vi "FRC Classification Example.vi"() -> ()   [LabVIEW 2025]
uses:
  <vilib>/Rock Robotics/WPI/Camera/WPI_CameraSettings Read MJPG.ctl
  <vilib>/Rock Robotics/WPI/Camera/WPI_CameraImageSize.ctl
  Vision Support Code/Camera Types.ctl
  <vilib>/vision/NI_Vision_Development_Module.lvlib
panel:
  in  "score limit":sgl
  in  "Limit Tests?":bool=TRUE
  in  "Camera Type":T1=enum."MS HD3000 square"
  in  "Image Path":path=path "Sample Images/KicoffFilmingVision"
  in  "image files":string[](array[string])
  in  "Aspect Fudge Factor":dbl=1.0
  out "Detected Targets":T2(array[cluster]) {"Normalized Rect"."Numeric 5" format="%#_2g"; "Normalized Rect"."Numeric 3" format="%#_2g"; "Normalized Rect"."Numeric 2" format="%#_2g"; "Normalized Rect"."Numeric" format="%#_2g"}
  in  "Score Threshold":dbl=75.0
  in  "Source":enum32{"Files", "Camera"}(tab)
  in  "Images":i32(listbox)
  in  "Folder Location":path=path "Sample Images/Real Tower"
  in  "Camera Settings":T3={"fps"=20, "compression"=30, "Image Size"=enum."320x240", "Config Shown"=FALSE}
  in  "Camera Address":string="USB 1"
  in  "Annotate":bool=TRUE
  out "ms to process":u32
  out "Sorted Scores":T5(array[cluster]) {"Moment Factor" format="%#_3g"; "L" format="%#_3g"; "Area to CH" format="%#_3g"; "X" format="%#_3g"; "Y" format="%#_3g"}
  in  "LED Color":T6={"Hue"={86.68604567358754, 144.18771039657545}, "Sat"={97.14285714285715, 255.0}, "Val"={39.46428571428572, 255.0}} {"Hue" scale=0.0..255.0 scale format="%#_3g"}
  out "Masked":T7(plugin-control)
  out "Original Image":T7(plugin-control)
  # "Instructions:\nUse Source to select image files from a directory, or use a USB or IP camera connected to your laptop.\nUse LED Color to threshold and build particles. Adjust HSV values to improve masking.\nAnnotations draw a rectangle around \"good\" particles with scores from top to bottom."
  # "Aspect Ratio"
  # "Density Profile"
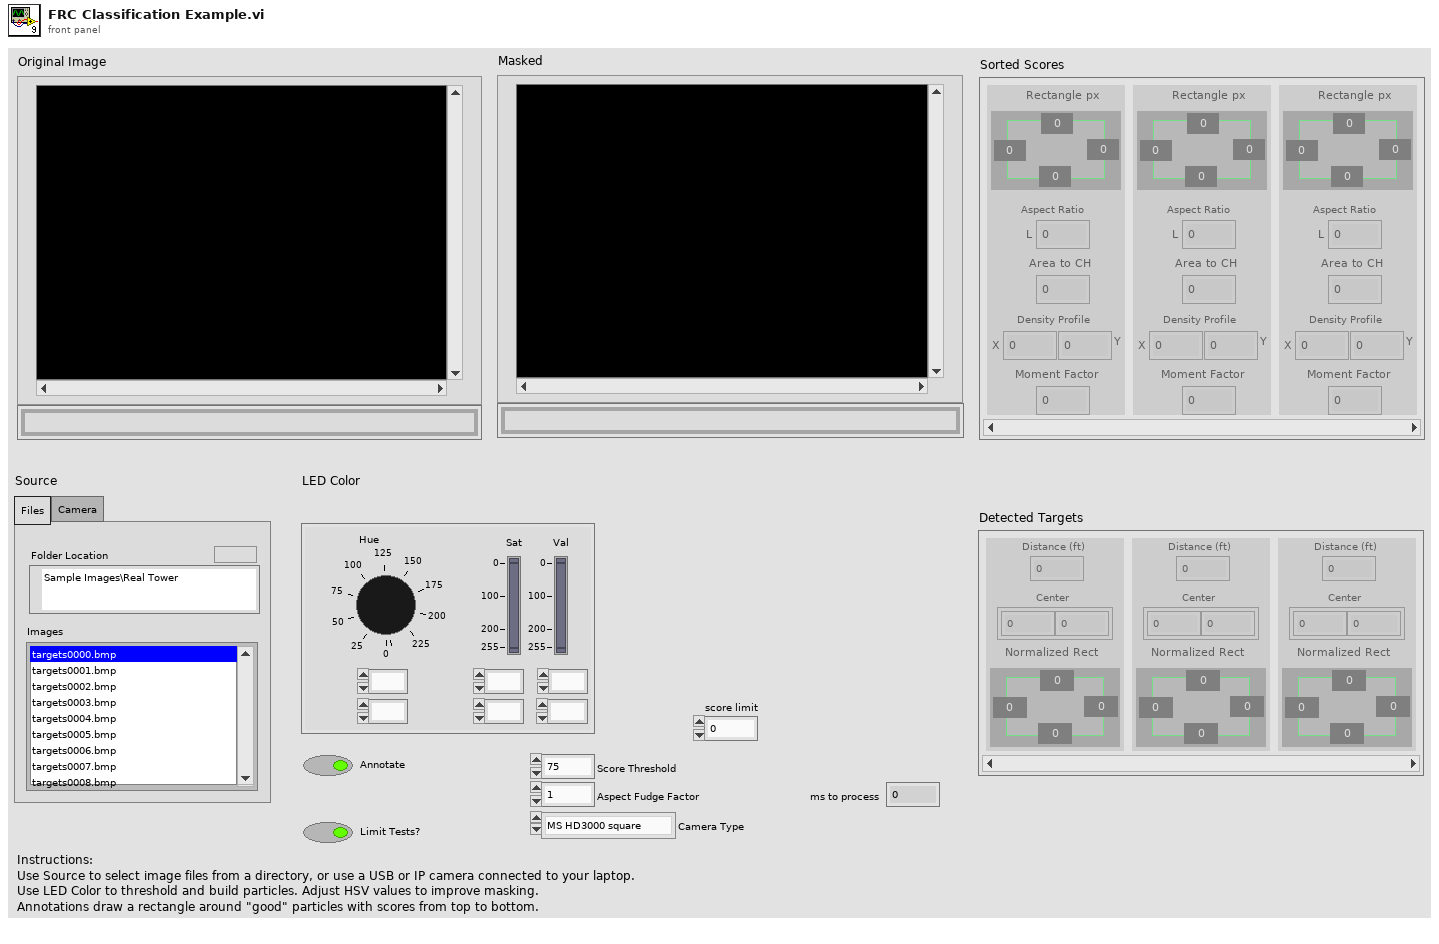
[diagram p1: front panel]
types:
  T1 = typedef "Camera Types.ctl" = enum16{"206", "1011", "1013", "MS HD3000 square", "MS HD3000 640x480"}
  T2 = cluster{"Distance (ft)":dbl, "Center":cluster{dbl, dbl}, "Normalized Rect":cluster{"Numeric":dbl, "Numeric 2":dbl, "Numeric 3":dbl, "Numeric 5":dbl}}[]
  T3 = typedef "WPI_CameraSettings Read MJPG.ctl" = cluster{"fps":i32, "compression":i32, "Image Size":T4, "Config Shown":bool}
  T4 = typedef "WPI_CameraImageSize.ctl" = enum16{"640x480", "320x240", "160x120", "Custom"}
  T5 = cluster{"Rectangle px":cluster{"Numeric":dbl, "Numeric 2":dbl, "Numeric 3":dbl, "Numeric 5":dbl}, "L":dbl, "Area to CH":dbl, "X":dbl, "Y":dbl, "Moment Factor":dbl}[]
  T6 = cluster{"Hue":cluster{dbl, dbl}, "Sat":cluster{dbl, dbl}, "Val":cluster{dbl, dbl}}
  T7 = typedef "IMAQ Image.ctl" = refnum<image>
  T8 = cluster{"Numeric":dbl, "Numeric":dbl, "Numeric":dbl, "Numeric":dbl, dbl}
  T9 = typedef "Image Type" = u32
  T10 = typedef "Particle Parameters" = i32
  T11 = typedef "IMAQ Classifier Session.ctl" = refnum<k1>
  T12 = typedef "ROI Descriptor" = cluster{"Global Rectangle":i32[], "Contours":cluster{"ID":enum32{"External", "Internal"}, "Type":u32, "Coordinates":i32[]}[]}
  T13 = cluster{"Classification Score":sgl, "Identification Score":sgl}
  T14 = cluster{"Numeric":dbl, "Numeric":dbl, "Numeric":dbl, "Numeric":dbl}
  T15 = cluster{"Rectangle":cluster{"Numeric":dbl, "Numeric 2":dbl, "Numeric 3":dbl, "Numeric 5":dbl}, "L":dbl, "Area to CH":dbl, "X":dbl, "Y":dbl, "Moment Factor":dbl}[]
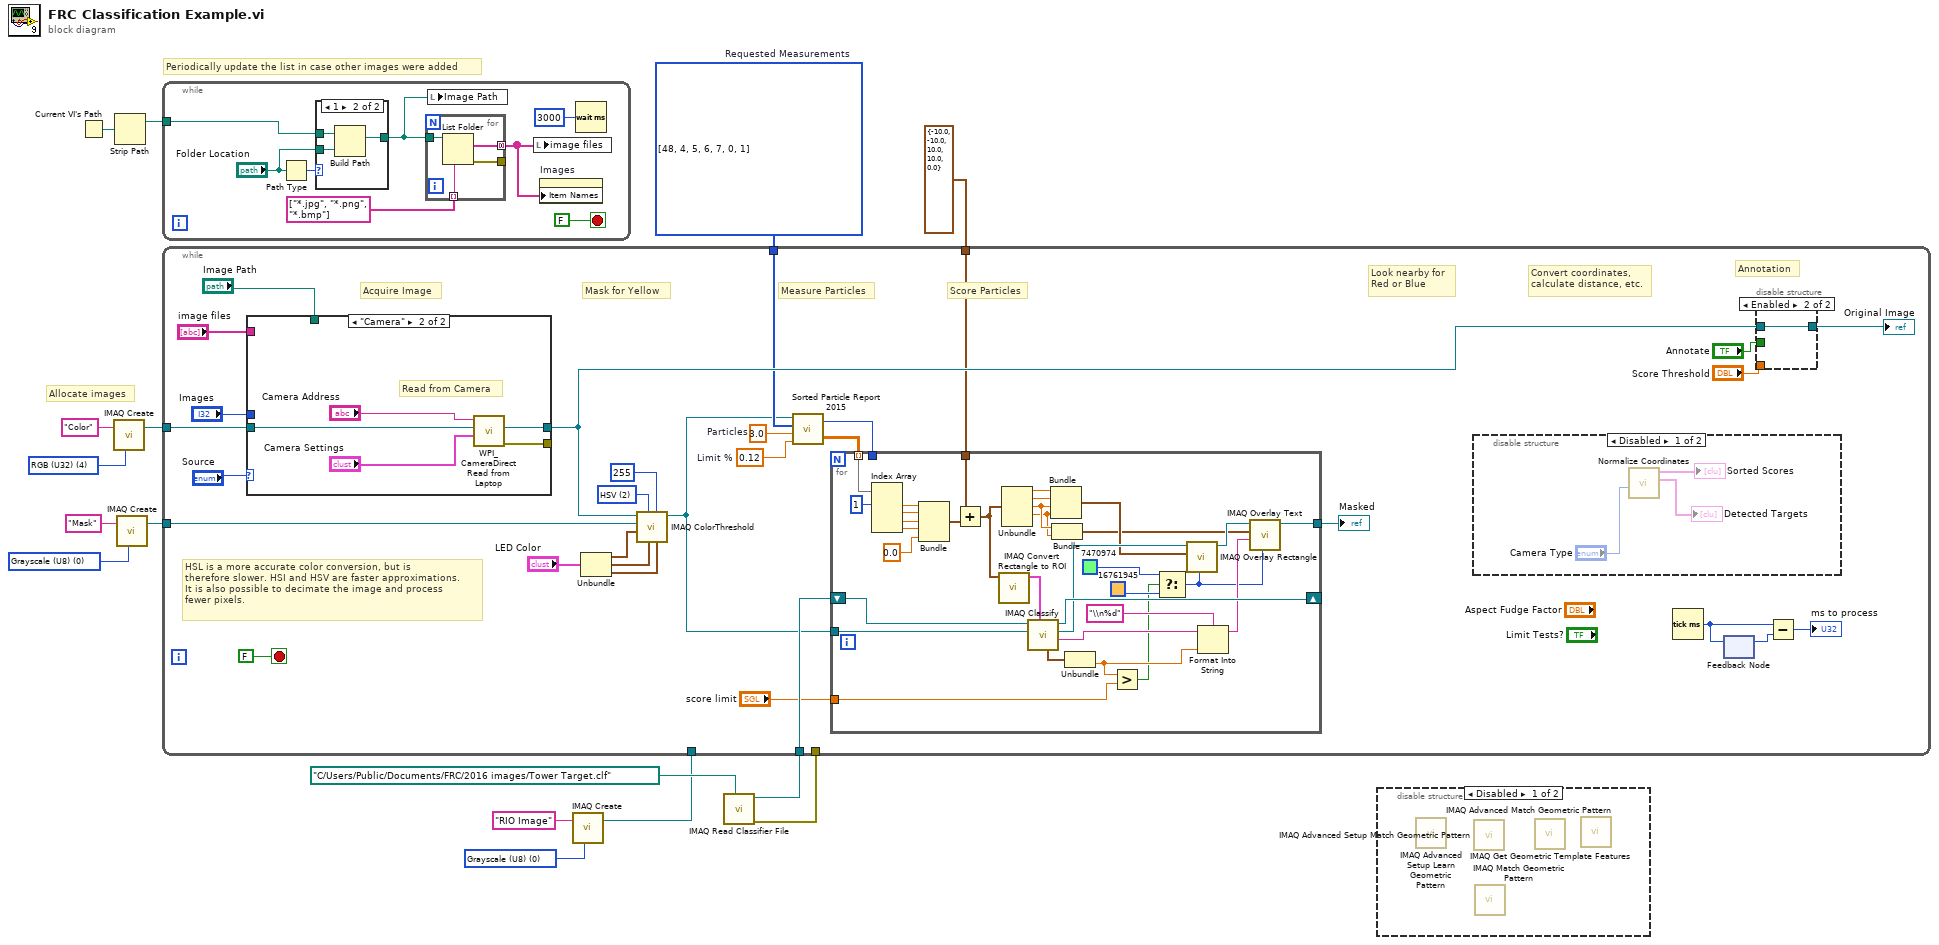
[diagram p0: block diagram]
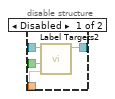
[diagram p4: hidden frame]
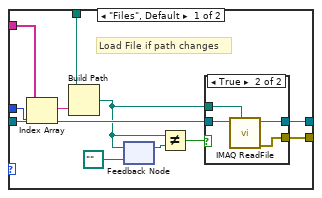
[diagram p6: hidden frame]
diagram:
  w4 = T9 0 items=["Grayscale (U8)", "Grayscale (I16)", "Grayscale (SGL)", "Complex (CSG)", "RGB (U32)", "HSL (U32)", "RGB (U64)", "Grayscale (U16)"] ("Image Type")
  w10 = T10[] [48, 4, 5, 6, 7, 0, 1] items=["Center of Mass X", "Center of Mass Y", "First Pixel X", "First Pixel Y", "Bounding Rect Left", "Bounding Rect Top", "Bounding Rect Right", "Bounding Rect Bottom", "Max Feret Diameter Start X", "Max Feret Diameter Start Y", "Max Feret Diameter End X", "Max Feret Diameter End Y", "Max Horiz. Segment Length Left", "Max Horiz. Segment Length Right", "Max Horiz. Segment Length Row", "-", "Bounding Rect Width", "Bounding Rect Height", "Bounding Rect Diagonal", "Perimeter", "Convex Hull Perimeter", "Holes' Perimeter", "Max Feret Diameter", "Equivalent Ellipse Major Axis", "Equivalent Ellipse Minor Axis", "Equivalent Ellipse Minor Axis (Feret)", "Equivalent Rect Long Side", "Equivalent Rect Short Side", "Equivalent Rect Diagonal", "Equivalent Rect Short Side (Feret)", "Average Horiz. Segment Length", "Average Vert. Segment Length", "Hydraulic Radius", "Waddel Disk Diameter", "-", "Area", "Holes' Area", "Particle & Holes' Area", "Convex Hull Area", "Image Area", "-", "Number of Holes", "Number of Horiz. Segments", "Number of Vert. Segments", "-", "Orientation", "Max Feret Diameter Orientation", "-", "% Area/Image Area", "% Area/(Particle & Holes' Area)", "Ratio of Equivalent Ellipse Axes", "Ratio of Equivalent Rect Sides", "-", "Elongation Factor", "Compactness Factor", "Heywood Circularity Factor", "Type Factor", "-", "Sum X", "Sum Y", "Sum XX", "Sum XY", "Sum YY", "Sum XXX", "Sum XXY", "Sum XYY", "Sum YYY", "-", "Moment of Inertia XX", "Moment of Inertia XY", "Moment of Inertia YY", "Moment of Inertia XXX", "Moment of Inertia XXY", "Moment of Inertia XYY", "Moment of Inertia YYY", "Norm. Moment of Inertia XX", "Norm. Moment of Inertia XY", "Norm. Moment of Inertia YY", "Norm. Moment of Inertia XXX", "Norm. Moment of Inertia XXY", "Norm. Moment of Inertia XYY", "Norm. Moment of Inertia YYY", "Hu Moment 1", "Hu Moment 2", "Hu Moment 3", "Hu Moment 4", "Hu Moment 5", "Hu Moment 6", "Hu Moment 7"]  # Requested Measurements
  w13 = T9 0 items=["Grayscale (U8)", "Grayscale (I16)", "Grayscale (SGL)", "Complex (CSG)", "RGB (U32)", "HSL (U32)", "RGB (U64)", "Grayscale (U16)"] ("Image Type")
  w15 = T9 4 items=["Grayscale (U8)", "Grayscale (I16)", "Grayscale (SGL)", "Complex (CSG)", "RGB (U32)", "HSL (U32)", "RGB (U64)", "Grayscale (U16)"] ("Image Type")
  # "Periodically update the list in case other images were added"
  # "Allocate images"
  n1 = Current VI's Path() -> (path=w9:path)
  n2 = call "IMAQ Create"("Image Name"="Color", "Image Type"=w15) -> ("New Image"=w14:T7)  [unwired: 2 in, 2 out]
  n3 = Strip Path(path=w9) -> (stripped path=w8:path)  [unwired: 1 out]
  n4 = call "IMAQ Create"("Image Name"="Mask", "Image Type"=w13) -> ("New Image"=w11:T7)  [unwired: 2 in, 2 out]
  n5 = while {
    tunnel: w8 -> [w19]
    stop <- FALSE stop-if-true
    n6 = Path Type(1:"Folder Location") -> (0:w21:i16)
    n7 = case shown="1" w21 {
      tunnel: "Folder Location" -> [w25 w28]
      tunnel: [w25 w26] -> w18
      tunnel: w19 -> [_ w27]
      frame 0, Default {
      }
      frame 1 {
        n8 = Build Path(base path=w27, name or relative path=w28) -> (appended path=w26:path)
      }
    }
    n9 = for {
      tunnel: [w32] -> w22 mode=concatenating
      tunnel: w18 -> [w31]
      tunnel: string[] ["*.jpg", "*.png", "*.bmp"] -> [w30] mode=indexing
      tunnel: [w29] -> _
      n10 = List Folder(path=w31, pattern=w30) -> (filenames=w32:string[], error out=w29:errorcluster)  [unwired: 2 in, 2 out]
    }
    n11 = local write "Image Path"(w18) -> ()
    n12 = local write "image files"(w22) -> ()
    n13 = property on="Images" class="LstBox (strict)"("Item Names"=w22) -> ()  [unwired: 2 in, 2 out]
    n14 = Wait (ms)(milliseconds to wait=u32 3000) -> ()  [unwired: 1 out]
  }
  n15 = call "IMAQ Create"("Image Name"="RIO Image", "Image Type"=w4) -> ("New Image"=w3:T7)  [unwired: 2 in, 2 out]
  n16 = call "IMAQ Read Classifier File"("File Path"=path "C:/Users/Public/Documents/FRC/2016 images/Tower Target.clf") -> ("error out"=w2:errorcluster, "Classifier Session"=w6:T11)  [unwired: 6 in, 3 out]
  n17 = while {
    tunnel: w14 -> [w61]
    tunnel: w11 -> [w60]
    tunnel: w10 -> [w41]
    tunnel: w6 -> [w44]
    tunnel: w3 -> [_]
    tunnel: w2 -> [_]
    tunnel: T8 {"Numeric"=-10.0, "Numeric"=-10.0, "Numeric"=10.0, "Numeric"=10.0, 0.0} ("x") -> [w38]
    stop <- FALSE stop-if-true
    w42 = 0.12  # Limit %
    w43 = 3.0  # Particles
    w59 = u16 2 items=["RGB", "HSL", "HSV", "HSI"] ("Color Mode")
    # "Measure Particles"
    # "Convert coordinates,\ncalculate distance, etc."
    # "Annotation"
    # "Score Particles"
    # "Mask for Yellow"
    # "Acquire Image"
    # "HSL is a more accurate color conversion, but is\ntherefore slower. HSI and HSV are faster approximations.\nIt is also possible to decimate the image and process\nfewer pixels."
    # "Look nearby for\nRed or Blue"
    n18 = case shown="\"Camera\"" "Source" {
      tunnel: [w113 w124] -> _
      tunnel: [w114 w123] -> w46
      tunnel: w61 -> [w112 w122]
      tunnel: "image files" -> [w104 _]
      tunnel: "Images" -> [w111 _]
      tunnel: "Image Path" -> [w109 _]
      frame "Files", Default {
        # "Load File if path changes"
        n19 = Index Array(array=w104, index=w111) -> (element=w110:string)
        n20 = Build Path(base path=w109, name or relative path=w110) -> (appended path=w105:path)
        n21 = feedback-in #1(w105) -> ()
        n22 = feedback #1(path "" ("appended path")) -> (w107:path)
        n23 = Not Equal?(x=w105, y=w107) -> (x != y?=w108:bool)
        n24 = case shown="True" w108 {
          tunnel: [w115 w119] -> w114
          tunnel: [_ w118] -> w113
          tunnel: w112 -> [w115 w117]
          tunnel: w105 -> [_ w116]
          frame False {
          }
          frame True {
            n25 = call "IMAQ ReadFile"("File Path"=w116, "Image"=w117) -> ("error out"=w118:errorcluster, "Image Out"=w119:T7)  [unwired: 5 in, 3 out]
          }
        }
      }
      frame "Camera" {
        # "Read from Camera"
        n26 = call <vilib>:"WPI_CameraDirect Read from Laptop.vi"("Camera Settings"="Camera Settings", "Image"=w122, "address"="Camera Address") -> ("error out"=w124:errorcluster, "Image Out"=w123:T7)  [unwired: 7 in]
      }
    }
    n27 = Unbundle("LED Color") -> ("Hue"=w58:cluster{dbl, dbl}, "Sat"=w57:cluster{dbl, dbl}, "Val"=w56:cluster{dbl, dbl})
    n28 = call "IMAQ ColorThreshold"("Blue or Luma or Val or Inten Range"=w56, "Replace Value"=255, "Green or Sat Range"=w57, "Color Mode"=w59, "Red or Hue Range"=w58, "Image Dst"=w60, "Image Src"=w46) -> ("Image Dst Out"=w40:T7)  [unwired: 3 in, 1 out]
    n29 = call "Sorted Particle Report 2015.vi"("Min Area Size %"=w42, "Particle Count Limit"=w43, "Pixel Measurements"=w41, "Image in"=w40) -> ("Sorted Data"=w39:dbl[][], "Particles"=w37:i32)
    n30 = for {
      tunnel: w40 -> [w102]
      shift-right: [w101] -> _
      shift-left: w44 -> [w103]
      tunnel: w39 -> [w99] mode=indexing
      tunnel: w38 -> [w91]
      tunnel: w37 -> [_]
      tunnel: [w84] -> w36
      tunnel: "score limit" -> [w72]
      n31 = Index Array(array=w99, index #1=1 ("index")) -> (element #1=w94:dbl, element #2=w95:dbl, element #3=w96:dbl, element #4=w97:dbl)  [unwired: 3 in]
      n32 = Bundle("Numeric"=w94, "Numeric"=w95, "Numeric"=w96, "Numeric"=w97, 0.0) -> (w92:T8)  [unwired: 1 in]
      n33 = Add(x=w91, y=w92) -> (x+y=w87:T8)
      n34 = call "IMAQ Convert Rectangle to ROI"("Rectangle"=w87) -> ("ROI Descriptor"=w100:T12)  [unwired: 1 in, 8 out]
      n35 = Unbundle(w87) -> ("Numeric"=w89:dbl, "Numeric"=w88:dbl, "Numeric"=w83:dbl, "Numeric"=w82:dbl)  [unwired: 1 out]
      n36 = call "IMAQ Classify"("ROI Descriptor"=w100, "Image"=w102, "Classifier Session"=w103) -> ("Class"=w80:string, "Image (dup)"=w90:T7, "Classifier Session (dup)"=w101:T11, "Scores"=w79:T13)  [unwired: 3 in, 2 out]
      n37 = Bundle("Numeric"=w89, "Numeric"=w88, "Numeric"=w83, "Numeric"=w82) -> (w86:T14)  [unwired: 1 in]
      n38 = Bundle("Numeric"=w83, "Numeric"=w82) -> (w81:cluster{"Numeric":dbl, "Numeric":dbl})  [unwired: 1 in]
      n39 = Unbundle(w79) -> ("Identification Score"=w73:sgl)  [unwired: 1 out]
      n40 = Greater?(x=w73, y=w72) -> (0:w71:bool)
      n41 = Select(t=u32 7470974 ("Text Color (black)"), s=w71, f=u32 16761945 ("Text Color (black)")) -> (s? t:f=w76:u32)
      n42 = call "IMAQ Overlay Rectangle"("Color"=w76, "Rectangle"=w86, "Image"=w90) -> ("Image Out"=w85:T7)  [unwired: 7 in, 1 out]
      n43 = Format Into String(format string="\\n%d", initial string=w80, w73) -> (resulting string=w78:string)  [unwired: 1 in, 1 out]
      n44 = call "IMAQ Overlay Text"("Text Color (black)"=w76, "String"=w78, "Origin"=w81, "Image"=w85) -> ("Image Out"=w84:T7)  [unwired: 6 in, 1 out]
    }
    "Masked" <- w36
    n45 = disable-structure shown="Disabled" {
      frame Disabled {
        n46 = call "Normalize Coordinates.vi"("Camera Type"="Camera Type") -> ("Found Targets"=→"Detected Targets":T2, "Sorted Scores"=→"Sorted Scores":T15)  [unwired: 9 in]
      }
      frame Enabled {
      }
    }
    n47 = Tick Count (ms)() -> (millisecond timer value=w53:u32)
    n48 = feedback-in #2(w53) -> ()
    n49 = feedback #2() -> (w54:u32)  [unwired: 1 in]
    n50 = disable-structure shown="Enabled" {
      disable-tunnel: [w66 w67] -> w51
      disable-tunnel: "Annotate" -> [w65 _]
      disable-tunnel: "Score Threshold" -> [w64 _]
      disable-tunnel: w46 -> [w63 w67]
      frame Disabled {
        n51 = call "Label Targets2.vi"("Score Threshold"=w64, "Annotate"=w65, "Image in"=w63) -> ("Image out"=w66:T7)  [unwired: 8 in]
      }
      frame Enabled {
      }
    }
    "Original Image" <- w51
    n52 = Subtract(x=w53, y=w54) -> (x-y=→"ms to process":u32)
  }
  n53 = disable-structure shown="Disabled" {
    frame Disabled {
      n54 = call "IMAQ Advanced Setup Learn Geometric Pattern"() -> ()  [unwired: 9 in, 2 out]
      n55 = call "IMAQ Advanced Setup Match Geometric Pattern"() -> ()  [unwired: 9 in, 2 out]
      n56 = call "IMAQ Match Geometric Pattern"() -> ()  [unwired: 8 in, 4 out]
      n57 = call "IMAQ Get Geometric Template Features"() -> ()  [unwired: 10 in, 2 out]
      n58 = call "IMAQ Advanced Match Geometric Pattern"() -> ()  [unwired: 7 in, 5 out]
    }
    frame Enabled {
    }
  }
